vi "FTW-ERR-ThrowGenericError.vi"(7 "Error Message":string, 11 "error in":errorcluster) -> (15 "error out":errorcluster)   [LabVIEW 2015]
uses:
  FTW-ERR-CallChain.vi
  FTW-ERR-NoErrorConstant.vi
  string/FTW-STR-ReplaceWhitespace.vi
  string/FTW-STR-Array-Delimit.vi
  FTW-ERR-Clear.vi
  regex/FTW-Regex-ReplaceAll.vi
panel:
  # "Inputs"
  # "Outputs"
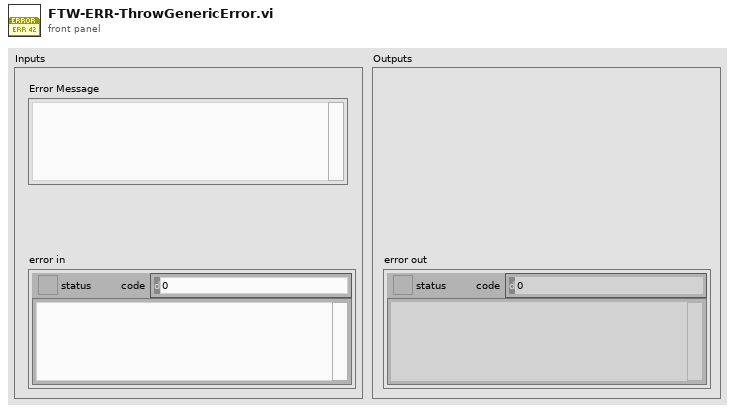
[diagram p1: front panel]
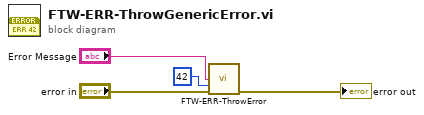
[diagram p0: block diagram]
diagram:
  n1 = call "FTW-ERR-ThrowError.vi"("Error Message"="Error Message", "Error Code"=42 ("code"), "error in"="error in") -> ("error out"=→"error out":errorcluster)  [unwired: 12 in]
